vi "Agilent DMM Get Stimulus.vi"(7 "Agilent DMM":T2, 8 "error in (no error)":errorcluster, 11 "VISA Resource Name":refnum<visa-resource-name>) -> (0 "error out":errorcluster, 2 "DCA Stimulus":T1, 3 "dup VISA Resource Name":refnum<visa-resource-name>)   [LabVIEW 2011]
uses:
  tests/DC Attenuation/TypeDefs/DCA Stimulus Parameters.ctl
  TypeDefs/Agilent DMM Instrument Info.ctl
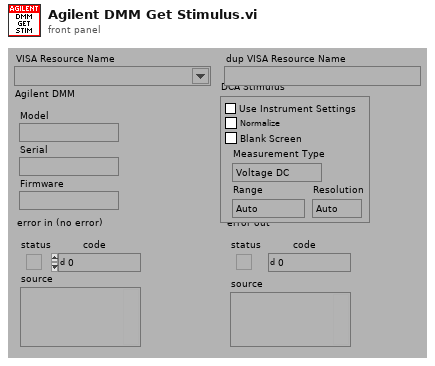
[diagram p1: front panel]
types:
  T1 = typedef "DCA Stimulus Parameters.ctl" = cluster{"Use Instrument":bool, "Normalize":bool, "Blank Screen":bool, "Measurement Type":enum16{"Voltage DC", "Voltage DC Ratio", "Voltage AC", "Current DC", "Current AC", "Resistance", "Fresistance", "Frequency", "Period", "Continuity", "Diode"}, "Range":enum16{"Auto", "Minimum", "Maximum", "100", "1,000", "10,000", "100,000", "1,000,000", "10,000,000", "100,000,000"}, "Resolution":enum16{"Auto", "4 1/2", "5 1/2", "6 1/2"}}
  T2 = typedef "Agilent DMM Instrument Info.ctl" = cluster{"Model":string, "Serial":string, "Firmware":string}
  T3 = typedef "Agilent DMM Measurement Type.ctl" = enum16{"Voltage DC", "Voltage DC Ratio", "Voltage AC", "Current DC", "Current AC", "Resistance", "Fresistance", "Frequency", "Period", "Continuity", "Diode"}
  T4 = typedef "Agilent DMM Range.ctl" = enum16{"Auto", "Min", "Max", "0.01", "0.1", "1", "3", "10", "100", "1,000", "10,000", "100,000", "1,000,000", "10,000,000", "100,000,000"}
  T5 = typedef "Agilent DMM Resolution.ctl" = enum16{"Auto", "Min", "Max", "4 1/2", "5 1/2", "6 1/2"}
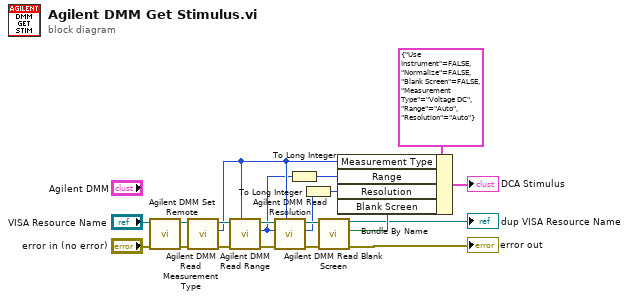
[diagram p0: block diagram]
diagram:
  n1 = call "Agilent DMM Set Remote.vi"("error in (no error)"="error in (no error)", "VISA Resource Name"="VISA Resource Name") -> ("error out"=w13:errorcluster, "dup VISA Resource Name"=w14:refnum<visa-resource-name>)  [unwired: 8 out]
  n2 = call "Agilent DMM Read Measurement Type.vi"("error in (no error)"=w13, "VISA Resource Name"=w14) -> ("error out"=w18:errorcluster, "Measurement Type"=w5:T3, "dup VISA Resource Name"=w17:refnum<visa-resource-name>)  [unwired: 7 out]
  n3 = call "Agilent DMM Read Range.vi"("Measurement Type"=w5, "error in (no error)"=w18, "VISA Resource Name"=w17) -> ("error out"=w12:errorcluster, "Range"=w4:T4, "dup VISA Resource Name"=w11:refnum<visa-resource-name>)  [unwired: 1 in, 5 out]
  n4 = call "Agilent DMM Read Resolution.vi"("Measurement Type"=w5, "error in (no error)"=w12, "Range"=w4, "VISA Resource Name"=w11) -> ("error out"=w10:errorcluster, "Resolution"=w2:T5, "dup VISA Resource Name"=w9:refnum<visa-resource-name>)  [unwired: 5 out]
  n5 = To Long Integer(number=w4) -> (32bit integer=w3:i32)
  n6 = To Long Integer(number=w2) -> (32bit integer=w1:i32)
  n7 = call "Agilent DMM Read Blank Screen.vi"("error in (no error)"=w10, "VISA Resource Name"=w9) -> ("error out"=→"error out":errorcluster, "Blank Screen"=w8:bool, "dup VISA Resource Name"=→"dup VISA Resource Name":refnum<visa-resource-name>)  [unwired: 7 out]
  n8 = Bundle By Name(cluster=T1 {"Use Instrument"=FALSE, "Normalize"=FALSE, "Blank Screen"=FALSE, "Measurement Type"=enum."Voltage DC", "Range"=enum."Auto", "Resolution"=enum."Auto"} ("Stimulus"), "Measurement Type"=w5, "Range"=w3, "Resolution"=w1, "Blank Screen"=w8) -> (→"DCA Stimulus":T1)
